vi "Horizontal Pointer Slide (Silver).vi"() -> ()   [LabVIEW 2012]
panel:
  in  "Horizontal Pointer Slide":dbl(slide) scale=0.0..10.0
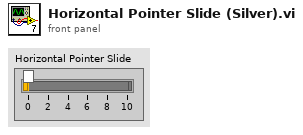
[diagram p1: front panel]
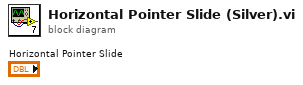
[diagram p0: block diagram]
diagram:
